vi "Global 1-Exp + IRF Convolution Fit v3.vi"(0 "Decays":cluster{"t Array":dbl[], "Data Array":dbl[]}[](array[cluster]), 1 "Initial Parameters":dbl[](array[numeric])=[-1.0, 0.0, 0.5, 0.1, 0.5, 1.0], 5 "Global Fit Parameters Info":T8={"Fit Data"=variant(cluster{"t Array":dbl[], "IRF Array":dbl[]} {"t Array"=[], "IRF Array"=[]}), "Global Fit Parameter Information"={"Original Parameter Indices"=[], "# Global Parameters"=0, "# Plot Specific Parameters"=0, "Global Parameter? Array"=[]}, "# Points in Plots"=[]}, 9 "Fit Options":T11={"Show Fit Residuals"=TRUE, "Fit Model"=enum."1-Exponential", "Residual Type"=enum."Standard", "Max Decay Percentile"=0.0, "Min Decay Percentile"=0.0, "Show Full Decay"=TRUE, "Weights"=enum."Unweighted", "Fitting Method"=enum."Least Square", "Compute Parameter Uncertainties"=TRUE, "Periodic Boundaries"=TRUE, "Model Calculation"=enum."Simulation", "Period"=1.2500000000000001e-08, "Termination Criteria"={"Max Iterations"=1000, "Max Function Calls"=0, "Max Time"=1000.0, "Function Tolerance"=1e-06, "Parameter Tolerance"=1e-06, "Gradient Tolerance"=0.0, "Min Lambda"=1e-06, "Max Lambda"=1e-06, "Initial Tick Count"=0}, "Offset Resolution"=1.2500000000000001e-08, "Use Local IRF"=TRUE, "Fitting Algorithm"=enum."Levenberg-Marquardt"} {"Offset Resolution" min=0.0; "Period" min=0.0; "Min Decay Percentile" min=0.0 max=1.0; "Max Decay Percentile" min=0.0 max=1.0}, 11 "error in (no error)":errorcluster, 12 "parameter bounds":T10, 13 "Termination Criteria":T1={"Max Iterations"=1000, "Max Function Calls"=10000, "Max Time"=1000.0, "Function Tolerance"=1e-06, "Parameter Tolerance"=1e-06, "Gradient Tolerance"=1e-06, "Min Lambda"=1e-06, "Max Lambda"=1e-06, "Initial Tick Count"=0}) -> (4 "Fitted Decays":cluster{"t Array":dbl[], "Fitted Array":dbl[]}[](array[cluster]), 6 "Residuals":T17(array[cluster]), 8 "Fit Output":T2={"best nonlinear fit"=[], "best fit parameters"=[], "R^2"=0.0, "RMSE"=0.0, "error out"={"status"=FALSE, "code"=0, "source"=""}, "Fitting Method"=enum."Least Square", "number of function calls"=0, "number of iterations"=0, "covariance"=[], "Chi 2"=0.0, "DOF"=0, "Fit Convergence Criterion"=enum."Continue", "Fitting Algorithm"=enum."Levenberg-Marquardt", "Weighted Fit"=FALSE, "Gradient"=0.0, "|Delta Chi 2|"=0.0, "|Delta Chi 2|/Chi 2"=0.0, "Max |Delta a| /|a|"=0.0, "Lambda"=-1.0, "RSS"=0.0, "AIC"=0.0, "BIC"=0.0, "Max number of function calls"=0, "Max number of iterations"=0, "IRF"={"X Array"=[], "Y Array"=[]}, "IRF Normalization Factor"=0.0, "Decay Normalization Factor"=0.0}, 10 "Delta Best Fit Parameters":dbl[](array[numeric]), 15 "error out":errorcluster)   [LabVIEW 2021]
uses:
  IRF(X)PSED/Decay Fit Options v2.ctl
  Decay Model.ctl
  Residual Type.ctl
  IRF(X)PSED/Fit Weights Type.ctl
  Non-linear Fitting Method v2.ctl
  Fit Calculation Method.ctl
  Non-linear Fitting Algorithm.ctl
  Global Fits/Global Fit Data.ctl
  Global Fits/Global Fit Parameters Information.ctl
  Non-linear Fit Output v3.ctl
  Nonlinear Fit Method.ctl
  <vilib>/Analysis/Matrix/Datatypes/RealMatrix.ctl
  Convergence Criteria.ctl
  Graphs/XY Graph/XY Plot Data.ctl
  My Fit Stopping Criteria.ctl
  AlliGator/AlliGator Settings List.ctl
  Fit Control Data.ctl
  <vilib>/Utility/error.llb/Error Cluster From Error Code.vi
  Global LM model function and gradient (1-Exp, Convolved, Periodic).vi
  <vilib>/ErrorRing/Error Ring.xnode
  Arrays/Arrays.lvlib
  Time/Time.lvlib
  Fits.lvlib
  Graphs/XY Graph/XY Graph Add-Ons.lvlib
  AlliGator/AlliGator Settings.lvlib
  <vilib>/Analysis/Matrix/NI_Matrix.lvlib
panel:
  out "CPU (s)":dbl
  out "XY Graph":T18(graph)
  # "Offset\nBaseline\nA1\ntau1"
  # "Offset\nBaseline\nA1\ntau 1\nA2\ntau 2"
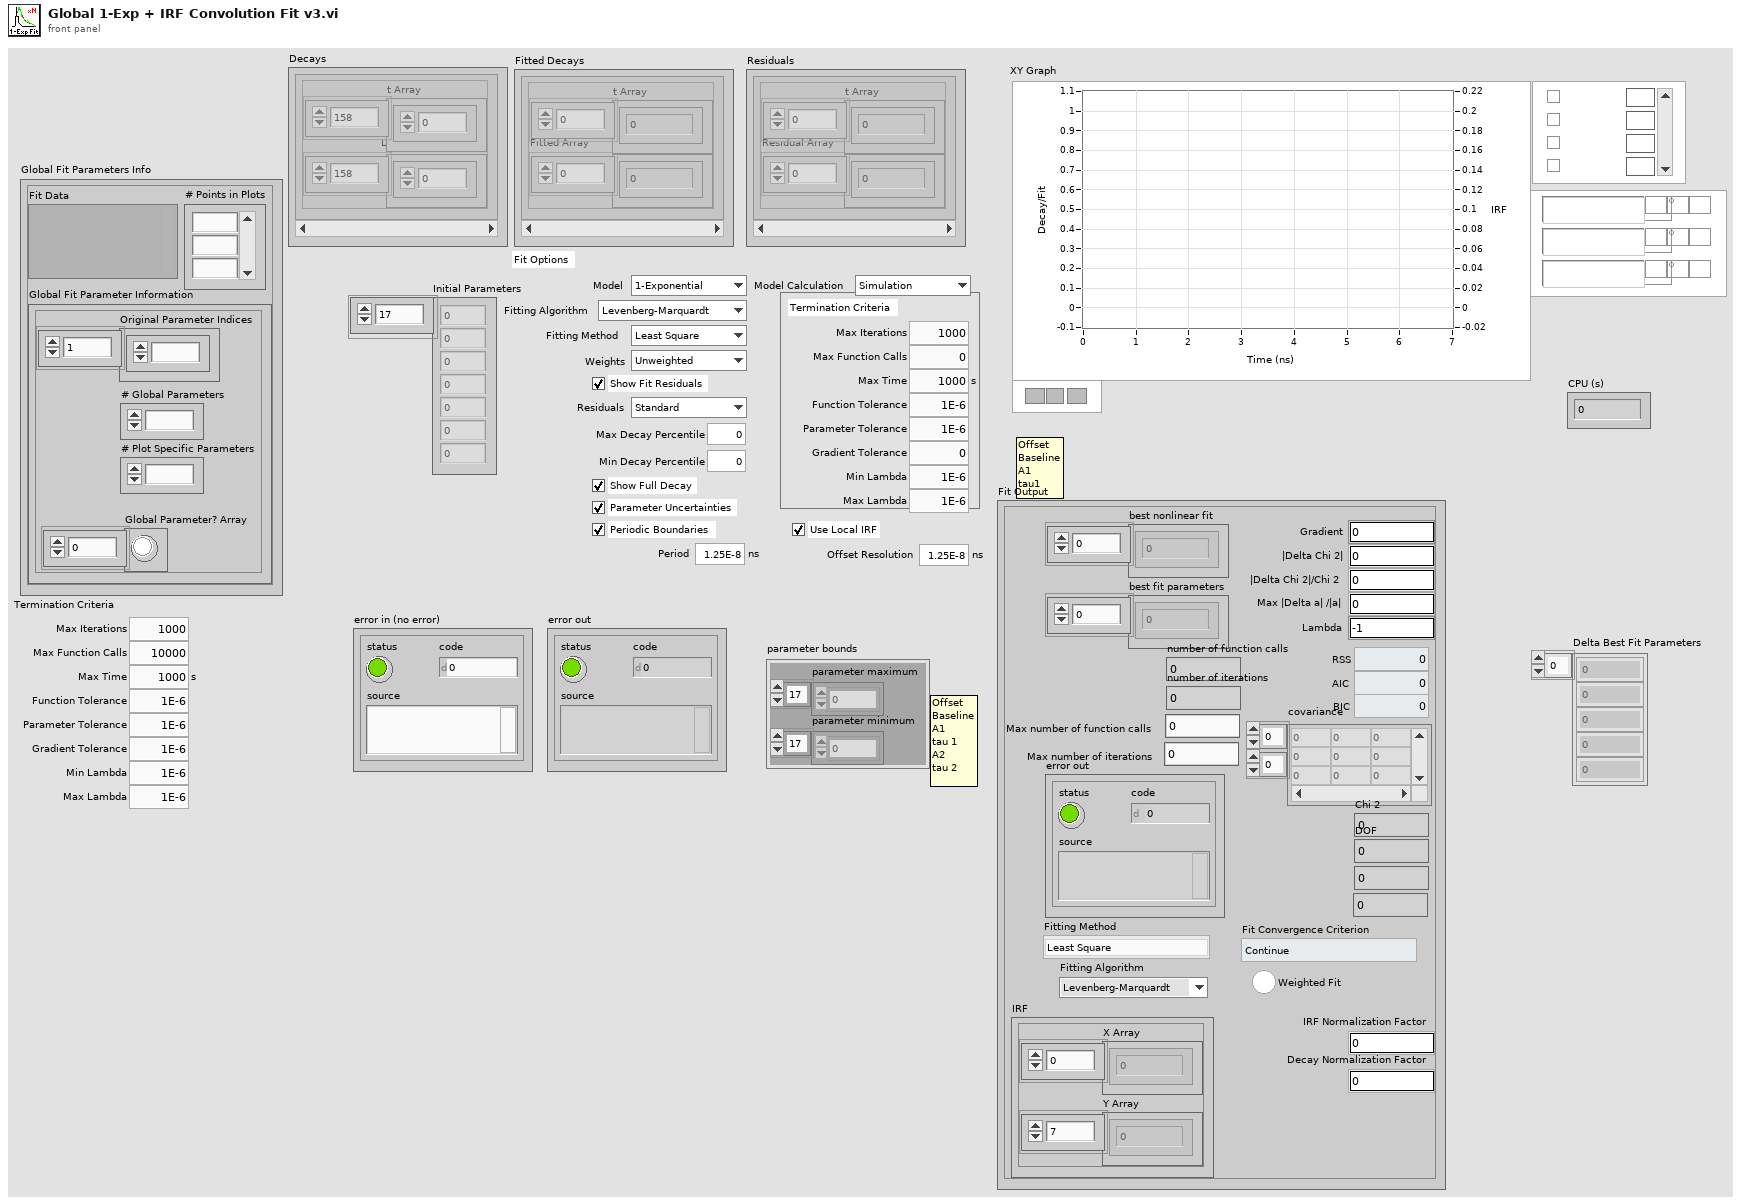
[diagram p1: front panel]
types:
  T1 = typedef "Fits.lvlib/My Fit Stopping Criteria.ctl" = cluster{"Max Iterations":i32, "Max Function Calls":i32, "Max Time":dbl[unit], "Function Tolerance":dbl, "Parameter Tolerance":dbl, "Gradient Tolerance":dbl, "Min Lambda":dbl, "Max Lambda":dbl, "Initial Tick Count":u32}
  T2 = typedef "Fits.lvlib/Non-linear Fit Output v3.ctl" = cluster{"best nonlinear fit":dbl[], "best fit parameters":dbl[], "R^2":dbl, "RMSE":dbl, "error out":errorcluster, "Fitting Method":T3, "number of function calls":i32, "number of iterations":i32, "covariance":T4, "Chi 2":dbl, "DOF":i32, "Fit Convergence Criterion":T5, "Fitting Algorithm":T6, "Weighted Fit":bool, "Gradient":dbl, "|Delta Chi 2|":dbl, "|Delta Chi 2|/Chi 2":dbl, "Max |Delta a| /|a|":dbl, "Lambda":dbl, "RSS":dbl, "AIC":dbl, "BIC":dbl, "Max number of function calls":i32, "Max number of iterations":i32, "IRF":T7, "IRF Normalization Factor":dbl, "Decay Normalization Factor":dbl}
  T3 = typedef "Fits.lvlib/Nonlinear Fit Method.ctl" = enum16{"Least Square", "Least Absolute Residual", "Bisquare", "MLE"}
  T4 = typedef "NI_Matrix.lvlib/RealMatrix.ctl" = dbl[][]
  T5 = typedef "Fits.lvlib/Convergence Criteria.ctl" = enum16{"Continue", "Tolerances Exceeded", "Max Time Exceeded", "Max Iterations Exceeded", "Max Function Evaluations Exceeded", "Scale Range Exceeded"}
  T6 = typedef "Fits.lvlib/Non-linear Fitting Algorithm.ctl" = enum16{"Levenberg-Marquardt", "Trust-Region Dogleg"}
  T7 = typedef "XY Graph Add-Ons.lvlib/XY Plot Data.ctl" = cluster{"X Array":dbl[], "Y Array":dbl[]}
  T8 = typedef "Global Fit Data.ctl" = cluster{"Fit Data":variant, "Global Fit Parameter Information":T9, "# Points in Plots":i32[]}
  T9 = typedef "Fits.lvlib/Global Fit Parameters Information.ctl" = cluster{"Original Parameter Indices":i32[], "# Global Parameters":i32, "# Plot Specific Parameters":i32, "Global Parameter? Array":bool[]}
  T10 = cluster{"parameter minimum":dbl[], "parameter maximum":dbl[]}
  T11 = typedef "Fits.lvlib/Decay Fit Options v2.ctl" = cluster{"Show Fit Residuals":bool, "Fit Model":T12, "Residual Type":T13, "Max Decay Percentile":dbl, "Min Decay Percentile":dbl, "Show Full Decay":bool, "Weights":T14, "Fitting Method":T15, "Compute Parameter Uncertainties":bool, "Periodic Boundaries":bool, "Model Calculation":T16, "Period":dbl[unit], "Termination Criteria":cluster{"Max Iterations":i32, "Max Function Calls":i32, "Max Time":dbl[unit], "Function Tolerance":dbl, "Parameter Tolerance":dbl, "Gradient Tolerance":dbl, "Min Lambda":dbl, "Max Lambda":dbl, "Initial Tick Count":u32}, "Offset Resolution":dbl[unit], "Use Local IRF":bool, "Fitting Algorithm":T6}
  T12 = typedef "Fits.lvlib/Decay Model.ctl" = enum16{"1-Exponential", "2-Exponentials"}
  T13 = typedef "Fits.lvlib/Residual Type.ctl" = enum16{"Standard", "Normalized", "Reduced"}
  T14 = typedef "Fits.lvlib/Fit Weights Type.ctl" = enum16{"Unweighted", "1/Variance", "Best of All"}
  T15 = typedef "Fits.lvlib/Non-linear Fitting Method v2.ctl" = enum16{"Least Square", "Least Absolute Residual", "Bisquare", "MLE", "-", "Best of All"}
  T16 = typedef "Fits.lvlib/Fit Calculation Method.ctl" = enum16{"Simulation", "Convolution", "Integration"}
  T17 = cluster{"t Array":dbl[], "Residual Array":dbl[]}[]
  T18 = cluster{"t Array":dbl[], "best nonlinear fit":dbl[]}[]
  T19 = typedef "AlliGator Settings.lvlib/AlliGator Settings List.ctl" = enum16{"GUI:Visible Settings Tab", "GUI:Last Run Version", "Source Image:Use Image Histogram for Contrast", "Source Image:Low Count Pixels Rejection Options", "Source Image:High Count Pixels Rejection Options", "Source Image:Use Image Brightness", "Source Image:Blend Overlay with Image Background", "Source Image:Use Fixed ROI Diameter", "Source Image:ROI Diameter", "Source Image:ROI Center Color", "Source Image:Peak Threshold", "Source Image:Intensity Threshold", "Source Image:Image Binning Options", "Source Image:Image Smoothing Options", "Source Image:Image Histogram Active", "Source Image:Invert Binary Mask", "Source Image:Hot Pixel Removal", "Source Image:Overlay Analyzed ROI Center", "Source Image:Auto-Adjust Contrast", "Source Image:Histogram Lower Percentile", "Source Image:Histogram Upper Percentile", "Source Image:Save Source Image", "Source Image:Scale Bar Options", "Source Image:Image Resolution (Pixel Size)", "Source Image:Flatfield Correction", "Data Information:Gate Width", "Data Information:Nanotime Gate Separation", "Data Information:Macrotime Gate Separation", "Data Information:Gate Step", "Data Information:# Gates", "Data Information:Gate Image Exposure", "Data Information:Gate Image Integration", "Data Information:Gates to Skip", "Data Information:Gates to Keep", "Data Information:Define Gates to", "Data Information:Channel Name", "Data Information:Available Channel Names", "Data Information:Channel Arithmetic", "Data Information:Background File Subtraction", "Data Information:Background File", "Data Information:Background Scaling Factor", "Data Information:Background Pile-up Correction", "Data Information:Background Pixel Well Capacity", "Data Information:Laser Period", "Data Information:SYNC Period", "Data Information:Pile-up Correction", "Data Information:Pixel Well Capacity", "Data Information:Dataset Scaling Factor", "Fluorescence Decay_Decay Pre-Processing:Reverse Gates", "Fluorescence Decay_Decay Pre-Processing:Verbose Decay Pre-Processing", "Fluorescence Decay_Decay Pre-Processing:Use Decay Pre-Processing", "Fluorescence Decay_Decay Pre-Processing:Background Subtraction", "Fluorescence Decay_Decay Pre-Processing:Background Definition Range", "Fluorescence Decay_Decay Pre-Processing:Baseline Subtraction Method", "Fluorescence Decay_Decay Pre-Processing:Operations Order", "Fluorescence Decay_Decay Pre-Processing:Smoothing Parameter", "Fluorescence Decay_Decay Pre-Processing:Shift Decay", "Fluorescence Decay_Decay Pre-Processing:Decay Shift Parameters", "Fluorescence Decay_Decay Pre-Processing:Fold Decay", "Fluorescence Decay_Decay Pre-Processing:# Folds", "Fluorescence Decay_Decay Pre-Processing:1-Normalize Decay", "Fluorescence Decay_Decay Pre-Processing:[0-1]-Normalize Decay", "Fluorescence Decay_Decay Pre-Processing:Smoothen Decay", "Fluorescence Decay_Decay Pre-Processing:Extrapolate Decay", "Fluorescence Decay_Decay Pre-Processing:Use Periodicity", "Fluorescence Decay_Decay Pre-Processing:Use Cursors", "Fluorescence Decay_Decay Pre-Processing:Tail Fraction", "Fluorescence Decay_Decay Pre-Processing:Head Fraction", "Fluorescence Decay_Decay Pre-Processing:Additional Points", "Fluorescence Decay_Decay Pre-Processing:Straighten Decay", "Fluorescence Decay_Decay Pre-Processing:Constant Background", "Fluorescence Decay_Decay Pre-Processing:Pixel-Normalize Decay", "Fluorescence Decay_Advanced Analysis:Extract IRF instead of Decay", "Fluorescence Decay_Advanced Analysis:IRF Extraction Options", "Fluorescence Decay_Advanced Analysis:IRF Optimization Options", "Fluorescence Decay_Advanced Analysis:Square Pulse Options", "Fluorescence Decay_Advanced Analysis:IRF Order", "Fluorescence Decay_Advanced Analysis:IRF Time Constants", "Fluorescence Decay_Advanced Analysis:Wavelet Analysis Options", "Fluorescence Decay_Advanced Analysis:Average Lifetime Options", "Fluorescence Decay_Fit Options:Fit Options", "Fluorescence Decay_Fit Options:Use Legacy Fitting Approach", "Fluorescence Decay_Fit Options:Use Data Information Laser Period", "Fluorescence Decay_Fit Parameters:Displayed Fit Parameters", "Fluorescence Decay_Fit Parameters:Fit Parameter Constraints", "Fluorescence Decay_Fit Parameters:Export Tabulated Results", "Fluorescence Decay_Fit Parameters:MLE Baseline Offset Type", "Fluorescence Decay_Fit Parameters:MLE Baseline Offset", "Fluorescence Decay_Fit Parameters:Guess Parameter Names", "Fluorescence Decay_Fit Parameters:Guess Parameter Values", "Fluorescence Decay_Fit Parameters:Guess Parameters Options", "Fluorescence Decay_Styles:Show Last Decay Only", "Fluorescence Decay_Styles:Decay Graph Color Array", "Fluorescence Decay:Decay Graph Active", "Fluorescence Decay Statistics:Min Peak Value", "Fluorescence Decay Statistics:Reject Low Decay Peak Pixels", "Fluorescence Decay Statistics:Reject High Decay Peak Pixels", "Fluorescence Decay Statistics:Max Peak Value", "Time Traces:Use File Timestamp", "Time Traces:Time Step", "Time Traces:Use Intensity Correction File", "Time Traces:Intensity Correction File", "Phasor Plot:Phasor Plot Smoothing Options", "Phasor Plot:Phasor Plot Size", "Phasor Plot:Phasor Plot Graphics Options", "Phasor Plot:Cumulative Phasor Plot", "Phasor Plot:Use Phasor Brightness", "Phasor Plot:Blend Overlay with Phasor Background", "Phasor Plot:Save Phasor Plot", "Phasor Plot:Show References", "Phasor Plot:Phasor Ratio Decay Range", "Phasor Plot:Exponential Fading", "Phasor Plot:Phasor Ratio Reference Colors", "Phasor Plot:Reference Radius", "Phasor Plot:Show Color Map Vertices", "Phasor Plot:Phasor Plot Active", "Phasor Plot:Phasor Ratio Color Map Type", "Phasor Plot:Phasor Ratio Color Map", "Phasor Plot:Phasor Ratio Display Range", "Phasor Plot:Selected Image ROI(s)", "Phasor Plot:All Image ROIs", "Phasor Plot:Selected Phasor Plot ROI(s)", "Phasor Plot:All Phasor Plot ROIs", "Phasor Plot:Phasor Ratio Color-Coded Quantity", "Phasor Plot:Store Phasor Harmonics", "Phasor Plot:Draw Reference Segment", "Phasor Plot:User-Defined Quantity", "Phasor Graph:Phasor Frequency", "Phasor Graph:Phasor Ratio Type", "Phasor Graph:Pixel-level Phasor Computation", "Phasor Graph:Save Phasor Graph", "Phasor Graph:Phasor Graph Active", "Phasor Graph:Phasor SDV Options", "Phasor Calibration:Use Backup Calibration if needed", "Phasor Graph:Define Shortest Lifetime as", "Phasor Calibration:Backup Calibration Type", "Phasor Calibration:Calibration Type", "Phasor Calibration:Calibration Lifetime", "Phasor Calibration:Calibration Map Algorithm", "Single-Exponential Phasor Locus (SEPL):Gate Parameters", "Single-Exponential Phasor Locus (SEPL):User-defined Gate", "Single-Exponential Phasor Locus (SEPL):User-defined IRF", "Single-Exponential Phasor Locus (SEPL):Phasor Parameters", "Single-Exponential Phasor Locus (SEPL):Decay & IRF Parameters", "Single-Exponential Phasor Locus (SEPL):Display Parameters", "Lifetime Analysis:Decay Analysis Parameters", "Lifetime Analysis:Lifetime Map Active", "Plugins:Python Settings", "Miscellaneous:Verbose Mode", "Miscellaneous:Beep after Script", "Miscellaneous:Saved Image File Format", "Miscellaneous:Exported Gate Image Settings", "Miscellaneous:Include Loading in Timing", "Miscellaneous:Verbose Settings Mode", "Miscellaneous:Histogram Options", "Miscellaneous:Beep on Error", "Miscellaneous:# Logical Processors Used", "Miscellaneous:ROI Description Max Characters", "Miscellaneous:Verbose Error Mode", "Miscellaneous:Transparent Mask Color"}
  T20 = typedef "Fits.lvlib/Fit Control Data.ctl" = cluster{"IRF":T7, "Laser Period":dbl, "SYNC Period":dbl}
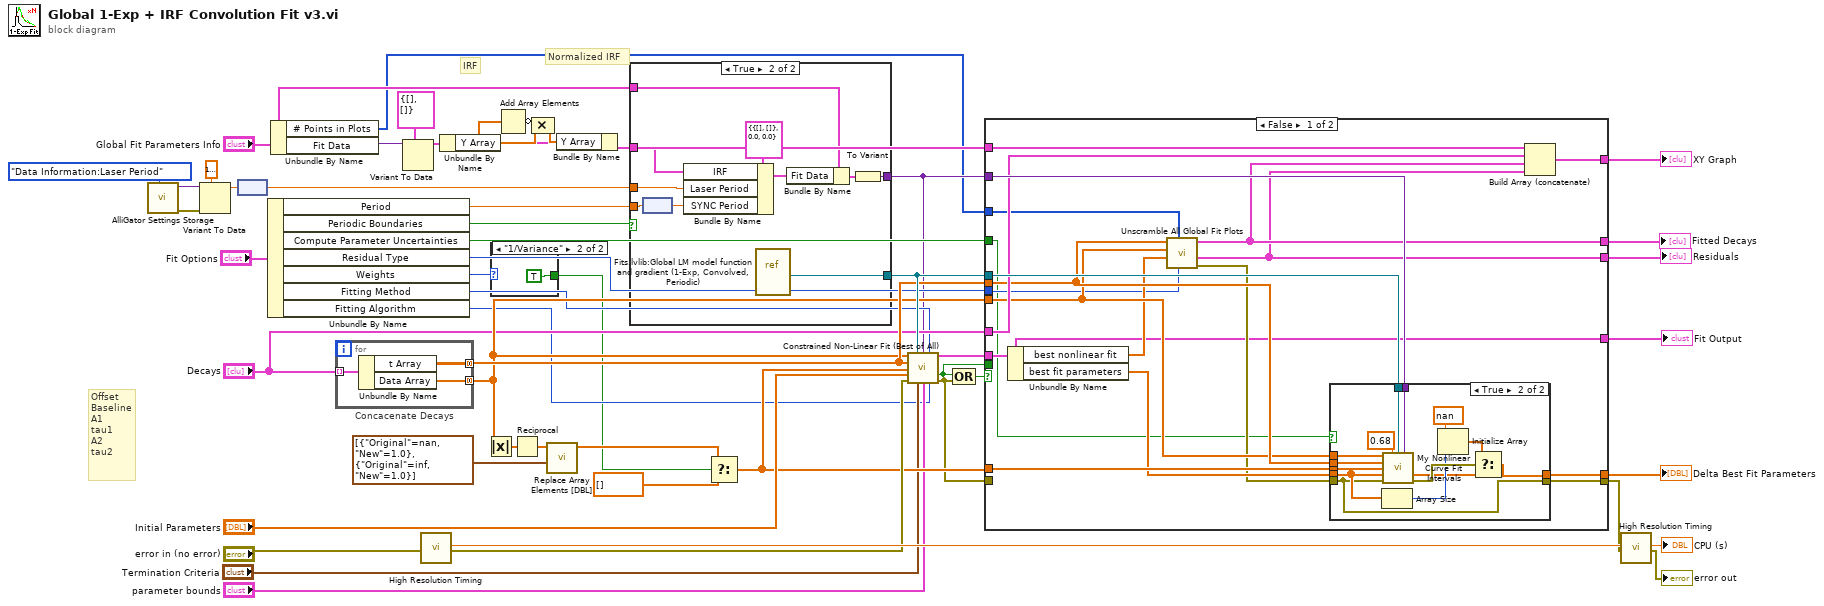
[diagram p0: block diagram]
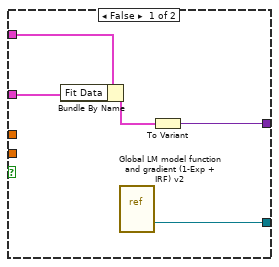
[diagram p3: hidden frame]
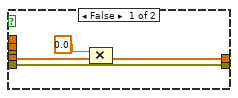
[diagram p4: hidden frame]
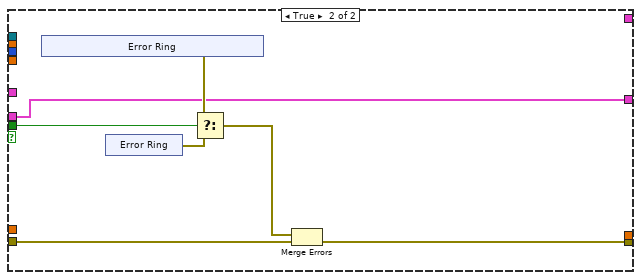
[diagram p5: hidden frame]
diagram:
  # "Normalized IRF"
  # "IRF"
  # "Offset\nBaseline\nA1\ntau1\nA2\ntau2"
  n1 = call "AlliGator Settings Storage.vi"("AlliGator Settings List"=AlliGator_Settings_List."Data Information:Laser Period") -> ("Error Out"=w8:errorcluster, "Variant Data out"=w9:variant)  [unwired: 9 in]
  n2 = Variant To Data(error in=w8, type=dbl[unit] 1e-09 ("New"), Variant=w9) -> (data=w6:dbl[unit])  [unwired: 1 out]
  n3 = node(w6) -> (w5:dbl)
  n4 = Unbundle By Name("Fit Options") -> ("Period"=w11:dbl[unit], "Periodic Boundaries"=w15:bool, "Compute Parameter Uncertainties"=w17:bool, "Residual Type"=w24:T13, "Weights"=w2:T14, "Fitting Method"=w19:T15, "Fitting Algorithm"=w3:T6)
  n5 = Unbundle By Name("Global Fit Parameters Info") -> ("# Points in Plots"=w4:i32[], "Fit Data"=w29:variant)
  n6 = for "Concacenate Decays" {
    tunnel: "Decays" -> [w56] mode=indexing
    tunnel: [w55] -> w26 mode=concatenating
    tunnel: [w54] -> w25 mode=concatenating
    n7 = Unbundle By Name(w56) -> ("t Array"=w55:dbl[], "Data Array"=w54:dbl[])
  }
  n8 = Variant To Data(type=T7 {"X Array"=[], "Y Array"=[]} ("Plot"), Variant=w29) -> (data=w27:T7)  [unwired: 1 in, 1 out]
  n9 = call "High Resolution Timing.vi"("Error In"="error in (no error)") -> ("elapsed (relative) seconds"=w48:dbl, "Error Out"=w39:errorcluster)  [unwired: 16 in, 1 out]
  n10 = Unbundle By Name(w27) -> ("Y Array"=w45:dbl[])
  n11 = Absolute Value(x=w25) -> (abs(x)=w53:dbl[])
  n12 = case shown="\"1/Variance\"" w2 {
    tunnel: [_ TRUE ("Weighted Fit")] -> w1
    frame "Unweighted", Default {
    }
    frame "1/Variance" {
    }
  }
  n13 = Add Array Elements(numeric array=w45) -> (sum=w46:dbl)
  n14 = Reciprocal(x=w53) -> (1/x=w52:dbl[])
  n15 = Compound Arithmetic op=MULTIPLY(invert w46, w45) -> (w44:dbl[])
  n16 = call "Replace Array Elements [DBL].vi"("Array of Replacement Pairs"=cluster{"Original":dbl, "New":dbl}[] [{"Original"=nan, "New"=1.0}, {"Original"=inf, "New"=1.0}], "Array"=w52) -> ("Array with Replacements"=w42:dbl[])  [unwired: 8 in, 1 out]
  n17 = Bundle By Name(cluster=w27, "Y Array"=w44) -> (w13:T7)
  n18 = case shown="True" w15 {
    tunnel: [w62 w67] -> w36
    tunnel: "Global Fit Parameters Info" -> [w61 w66]
    tunnel: w13 -> [w60 w71]
    tunnel: [w58 w63] -> w12
    tunnel: w11 -> [_ w69]
    tunnel: w5 -> [_ w70]
    frame False {
      n19 = Bundle By Name(cluster=w61, "Fit Data"=w60) -> (w59:T8)
      n20 = vi-ref "Global LM model function and gradient (1-Exp + IRF) v2.vi"() -> (w62:refnum<vi>)
      n21 = To Variant(anything=w59) -> (Variant=w58:variant)
    }
    frame True {
      n22 = node(w69) -> (w68:dbl)
      n23 = Bundle By Name(cluster=T20 {"IRF"={"X Array"=[], "Y Array"=[]}, "Laser Period"=0.0, "SYNC Period"=0.0} ("Fit Control Data"), "IRF"=w71, "Laser Period"=w70, "SYNC Period"=w68) -> (w65:T20)
      n24 = vi-ref "Fits.lvlib:Global LM model function and gradient (1-Exp, Convolved, Periodic).vi"() -> (w67:refnum<vi>)
      n25 = Bundle By Name(cluster=w66, "Fit Data"=w65) -> (w64:T8)
      n26 = To Variant(anything=w64) -> (Variant=w63:variant)
    }
  }
  n27 = Select(t=w42, s=w1, f=dbl[] [] ("Array with Replacements")) -> (s? t:f=w37:dbl[])
  n28 = call "Constrained Non-Linear Fit (Best of All).vi"("Y Array"=w25, "f(x,a)"=w36, "Data"=w12, "Fitting Method"=w19, "X Array"=w26, "Weights"=w37, "Guess Fitted Parameters"="Initial Parameters", "error in (no error)"=w39, "Termination Criteria"="Termination Criteria", "Fitted parameter bounds"="parameter bounds", "Fitting Algorithm"=w3) -> ("Fit Output"=w38:T2, "Fit Aborted?"=w20:bool, "Error Out"=w21:errorcluster)  [unwired: 1 in, 1 out]
  n29 = Compound Arithmetic op=OR(w20, w21) -> (w22:bool)
  n30 = case shown="False" w22 {
    tunnel: [w90 _] -> w35
    tunnel: [w77 _] -> w34
    tunnel: [w89 w112] -> w31
    tunnel: [w88 _] -> w32
    tunnel: [w76 _] -> w33
    tunnel: w24 -> [w79 _]
    tunnel: w26 -> [w82 _]
    tunnel: w25 -> [w81 _]
    tunnel: w37 -> [w87 _]
    tunnel: w13 -> [w83 _]
    tunnel: w38 -> [w75 w110]
    tunnel: w36 -> [w85 _]
    tunnel: "Decays" -> [w84 _]
    tunnel: w12 -> [w91 _]
    tunnel: w21 -> [_ w116]
    tunnel: w20 -> [_ w114]
    tunnel: [w75 w110] -> w18
    tunnel: w17 -> [w74 _]
    tunnel: w4 -> [w73 _]
    frame False {
      n31 = Unbundle By Name(w75) -> ("best nonlinear fit"=w80:dbl[], "best fit parameters"=w86:dbl[])
      n32 = call "Unscramble All Global Fit Plots.vi"("Residual Type"=w79, "# Points in Plots"=w73, "Best Nonlinear Fit Array"=w80, "Y array"=w81, "t Array"=w82) -> ("Error Out"=w78:errorcluster, "Decay Residuals"=w76:cluster{"Array":dbl[], "Array":dbl[]}[], "Fitted Decays"=w77:cluster{"Array":dbl[], "Array":dbl[]}[])  [unwired: 4 in]
      n33 = case shown="True" w74 {
        tunnel: w91 -> [_ w109]
        tunnel: [w95 w96] -> w89
        tunnel: [w93 w97] -> w88
        tunnel: w87 -> [_ w107]
        tunnel: w86 -> [w94 w99]
        tunnel: w85 -> [_ w106]
        tunnel: w82 -> [_ w105]
        tunnel: w81 -> [_ w104]
        tunnel: w78 -> [w95 w96]
        frame False {
          n34 = Compound Arithmetic op=MULTIPLY(0.0, w94) -> (w93:dbl[])
        }
        frame True {
          n35 = Array Size(array=w99) -> (size(s)=w100:i32)
          n36 = call "My Nonlinear Curve Fit Intervals.vi"("Y"=w104, "confidence level"=0.68, "f(x,a)"=w106, "data"=w109, "X"=w105, "Weight"=w107, "best fit parameters"=w99, "error in (no error)"=w96) -> ("delta best fit parameters"=w98:dbl[], "error out"=w103:errorcluster)  [unwired: 6 in]
          n37 = Initialize Array(nan ("element"), w100) -> (w102:dbl[])
          n38 = Select(t=w102, s=w103, f=w98) -> (s? t:f=w97:dbl[])
        }
      }
      n39 = Build Array (concatenate)(w83, w84, w77, w76) -> (w90:T7[])
    }
    frame True {
      n40 = xnode "Error Ring"() -> ("error out"=w113:errorcluster)
      n41 = xnode "Error Ring"() -> ("error out"=w115:errorcluster)
      n42 = Select(t=w113, s=w114, f=w115) -> (s? t:f=w111:errorcluster)
      n43 = Merge Errors(w111, w116) -> (w112:errorcluster)
    }
  }
  "Fitted Decays" <- w34
  "XY Graph" <- w35
  "Delta Best Fit Parameters" <- w32
  "Residuals" <- w33
  "Fit Output" <- w18
  n44 = call "High Resolution Timing.vi"("relative seconds (NaN)"=w48, "Error In"=w31) -> ("elapsed (relative) seconds"=→"CPU (s)":dbl, "Error Out"=→"error out":errorcluster)  [unwired: 15 in, 1 out]
